vi "DOCK_REPORT_CBATCH_get_data_from_SQL.vi"(8 "error_in":errorcluster, 11 "cbatch_code":string) -> (0 "error_out":errorcluster, 3 "SQL_result":variant, 4 "executed_SQL_statement":string)   [LabVIEW 2019]
uses:
  FGV/SQL_connection/FGV_DOCK_SQL_connection.ctl
  FGV/DOCK_REPORT_records_display/FGV_DOCK_REPORT_records_display.ctl
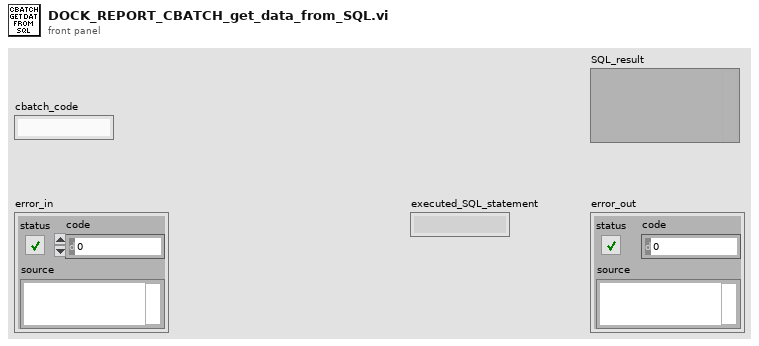
[diagram p1: front panel]
types:
  T1 = typedef "FGV_DOCK_REPORT_records_display.ctl" = enum16{"initialize", "set_cbatch_code", "set_records", "display", "clear", "get_all_info"}
  T2 = typedef "FGV_DOCK_SQL_connection.ctl" = enum16{"initialize", "connect", "read_tables", "read_columns", "SELECT", "INSERT", "UPDATE", "DELETE", "EXEC + headers", "EXEC", "TRANSACTION", "connection_active?", "disconnect"}
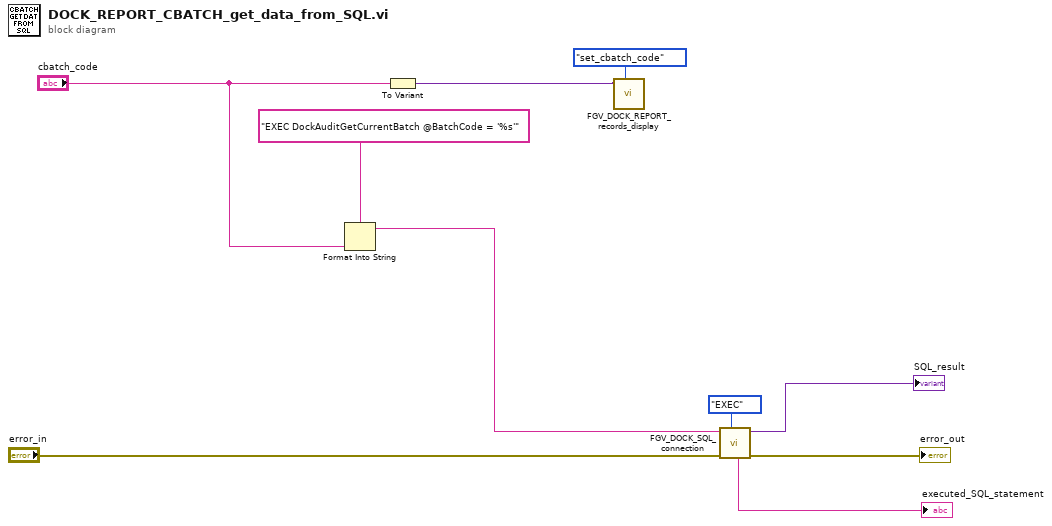
[diagram p0: block diagram]
diagram:
  n1 = Format Into String(format string="EXEC DockAuditGetCurrentBatch @BatchCode = '%s'", "cbatch_code") -> (resulting string=w4:string)  [unwired: 2 in, 1 out]
  n2 = To Variant(anything="cbatch_code") -> (Variant=w1:variant)
  n3 = call "FGV_DOCK_REPORT_records_display.vi"("options"=FGV_DOCK_REPORT_records_display."set_cbatch_code", "input"=w1) -> ()  [unwired: 8 in, 2 out]
  n4 = call "FGV_DOCK_SQL_connection.vi"("options"=FGV_DOCK_SQL_connection."EXEC", "error_in"="error_in", "SQL_statement"=w4) -> ("error_out"=→"error_out":errorcluster, "SQL_result"=→"SQL_result":variant, "executed_SQL_statement"=→"executed_SQL_statement":string)  [unwired: 4 in, 2 out]
